vi "PK camera tester CW viewer (frame trigger optional).vi"() -> ()   [LabVIEW 2018]
uses:
  <vilib>/userdefined/High Color/IMAQdx.ctl
  <vilib>/vision/driver/IMAQdx.llb/IMAQdx Attribute Type.ctl
  <vilib>/vision/driver/IMAQdx.llb/IMAQdx Buffer Number Mode.ctl
  convert 1D image array to 2D image - U8 input.vi
  <vilib>/Utility/file.llb/Write Delimited Spreadsheet (I64).vi
  <vilib>/vision/driver/NI_Vision_Acquisition_Software.lvlib
  <resource>/objmgr/imaqdx.rc
  <vilib>/vision/NI_Vision_Development_Module.lvlib
panel:
  out "frame time (s)":dbl format="%#_8g"
  out "frame rate (Hz)":dbl
  in  "stop":bool
  in  "filename":string="myImage"
  in  "path":path=path "C:/Users/QDM2exp/Documents/PK/LabView dev/pk camera stuff"
  in  "save?":bool
  out "max value":u8=131
  in  "external frame start triggers?":bool
  in  "Offset Y":i64(slide) min=0 max=1196 step=4 scale=0.0..1196.0
  in  "Offset X":i64(slide) min=0 max=1916 step=4 scale=0.0..1916.0
  in  "Width":i64(slide)=1920 min=0 max=1920 step=4 scale=0.0..1920.0
  in  "Height":i64(slide)=1200 min=0 max=1200 step=4 scale=0.0..1200.0
  out "Intensity Graph":u8[][](graph)
  in  "Exposure time (us)":dbl=6000.0 min=40.0 max=3000.0 step=1.0
  out "Attribute Information Array":T2(array[cluster])=[{"Attribute Type"=enum."U32", "Readable"=TRUE, "Writable"=TRUE, "Attribute Name"="AcquisitionAttributes::AdvancedGenicam::CommandTimeout"}, {"Attribute Type"=enum."U32", "Readable"=TRUE, "Writable"=TRUE, "Attribute Name"="AcquisitionAttributes::AdvancedGenicam::EventQueueDepth"}, {"Attribute Type"=enum."Bool", "Readable"=TRUE, "Writable"=TRUE, "Attribute Name"="AcquisitionAttributes::AdvancedGenicam::EventsEnabled"}, {"Attribute Type"=enum."Bool", "Readable"=TRUE, "Writable"=FALSE, "Attribute Name"="AcquisitionAttributes::AdvancedGenicam::EventsSupported"}, {"Attribute Type"=enum."Bool", "Readable"=TRUE, "Writable"=TRUE, "Attribute Name"="AcquisitionAttributes::AdvancedGenicam::IgnoreCameraValidationErrors"}, {"Attribute Type"=enum."U32", "Readable"=TRUE, "Writable"=FALSE, "Attribute Name"="AcquisitionAttributes::AdvancedUSB3Vision::ActualMaximumPayloadTransferSize"}, {"Attribute Type"=enum."U32", "Readable"=TRUE, "Writable"=FALSE, "Attribute Name"="AcquisitionAttributes::AdvancedUSB3Vision::RequiredPayloadSizeAlignment"}, {"Attribute Type"=enum."Enum", "Readable"=TRUE, "Writable"=TRUE, "Attribute Name"="AcquisitionAttributes::Bayer::Algorithm"}, {"Attribute Type"=enum."DBL", "Readable"=TRUE, "Writable"=TRUE, "Attribute Name"="AcquisitionAttributes::Bayer::GainB"}, {"Attribute Type"=enum."DBL", "Readable"=TRUE, "Writable"=TRUE, "Attribute Name"="AcquisitionAttributes::Bayer::GainG"}, {"Attribute Type"=enum."DBL", "Readable"=TRUE, "Writable"=TRUE, "Attribute Name"="AcquisitionAttributes::Bayer::GainR"}, {"Attribute Type"=enum."Enum", "Readable"=TRUE, "Writable"=TRUE, "Attribute Name"="AcquisitionAttributes::Bayer::Pattern"}, {"Attribute Type"=enum."Bool", "Readable"=TRUE, "Writable"=TRUE, "Attribute Name"="AcquisitionAttributes::ChunkDataDecoding::ChunkDataDecodingEnabled"}, {"Attribute Type"=enum."U32", "Readable"=TRUE, "Writable"=TRUE, "Attribute Name"="AcquisitionAttributes::ChunkDataDecoding::MaximumChunkCopySize"}, {"Attribute Type"=enum."Enum", "Readable"=TRUE, "Writable"=TRUE, "Attribute Name"="CameraAttributes::SequencerControl::SequencerMode"}, {"Attribute Type"=enum."I64", "Readable"=FALSE, "Writable"=FALSE, "Attribute Name"="CameraAttributes::SequencerControl::SequencerSetActive"}, {"Attribute Type"=enum."Enum", "Readable"=TRUE, "Writable"=TRUE, "Attribute Name"="CameraAttributes::SequencerControl::SequencerConfigurationMode"}, {"Attribute Type"=enum."I64", "Readable"=TRUE, "Writable"=FALSE, "Attribute Name"="CameraAttributes::SequencerControl::SequencerSetStart"}, {"Attribute Type"=enum."I64", "Readable"=TRUE, "Writable"=FALSE, "Attribute Name"="CameraAttributes::SequencerControl::SequencerSetSelector"}, {"Attribute Type"=enum."Command", "Readable"=FALSE, "Writable"=FALSE, "Attribute Name"="CameraAttributes::SequencerControl::SequencerSetLoad"}, {"Attribute Type"=enum."Command", "Readable"=FALSE, "Writable"=FALSE, "Attribute Name"="CameraAttributes::SequencerControl::SequencerSetSave"}, {"Attribute Type"=enum."I64", "Readable"=TRUE, "Writable"=FALSE, "Attribute Name"="CameraAttributes::SequencerControl::SequencerPathSelector"}, {"Attribute Type"=enum."I64", "Readable"=TRUE, "Writable"=FALSE, "Attribute Name"="CameraAttributes::SequencerControl::SequencerSetNext"}, {"Attribute Type"=enum."Enum", "Readable"=TRUE, "Writable"=FALSE, "Attribute Name"="CameraAttributes::SequencerControl::SequencerTriggerSource"}, {"Attribute Type"=enum."Enum", "Readable"=TRUE, "Writable"=FALSE, "Attribute Name"="CameraAttributes::SequencerControl::SequencerTriggerActivation"}, {"Attribute Type"=enum."I64", "Readable"=TRUE, "Writable"=FALSE, "Attribute Name"="CameraAttributes::ImageFormatControl::SensorWidth"}, {"Attribute Type"=enum."I64", "Readable"=TRUE, "Writable"=FALSE, "Attribute Name"="CameraAttributes::ImageFormatControl::SensorHeight"}, {"Attribute Type"=enum."I64", "Readable"=TRUE, "Writable"=FALSE, "Attribute Name"="CameraAttributes::ImageFormatControl::WidthMax"}, {"Attribute Type"=enum."I64", "Readable"=TRUE, "Writable"=FALSE, "Attribute Name"="CameraAttributes::ImageFormatControl::HeightMax"}, {"Attribute Type"=enum."I64", "Readable"=TRUE, "Writable"=TRUE, "Attribute Name"="CameraAttributes::ImageFormatControl::Width"}, {"Attribute Type"=enum."I64", "Readable"=TRUE, "Writable"=TRUE, "Attribute Name"="CameraAttributes::ImageFormatControl::Height"}, {"Attribute Type"=enum."I64", "Readable"=TRUE, "Writable"=TRUE, "Attribute Name"="CameraAttributes::ImageFormatControl::OffsetX"}, {"Attribute Type"=enum."I64", "Readable"=TRUE, "Writable"=TRUE, "Attribute Name"="CameraAttributes::ImageFormatControl::OffsetY"}, {"Attribute Type"=enum."Bool", "Readable"=TRUE, "Writable"=TRUE, "Attribute Name"="CameraAttributes::ImageFormatControl::CenterX"}, {"Attribute Type"=enum."Bool", "Readable"=TRUE, "Writable"=TRUE, "Attribute Name"="CameraAttributes::ImageFormatControl::CenterY"}, {"Attribute Type"=enum."Enum", "Readable"=TRUE, "Writable"=TRUE, "Attribute Name"="CameraAttributes::ImageFormatControl::BinningHorizontalMode"}, {"Attribute Type"=enum."I64", "Readable"=TRUE, "Writable"=TRUE, "Attribute Name"="CameraAttributes::ImageFormatControl::BinningHorizontal"}, {"Attribute Type"=enum."Enum", "Readable"=TRUE, "Writable"=TRUE, "Attribute Name"="CameraAttributes::ImageFormatControl::BinningVerticalMode"}, {"Attribute Type"=enum."I64", "Readable"=TRUE, "Writable"=TRUE, "Attribute Name"="CameraAttributes::ImageFormatControl::BinningVertical"}, {"Attribute Type"=enum."Bool", "Readable"=TRUE, "Writable"=TRUE, "Attribute Name"="CameraAttributes::ImageFormatControl::ReverseX"}, {"Attribute Type"=enum."Bool", "Readable"=TRUE, "Writable"=TRUE, "Attribute Name"="CameraAttributes::ImageFormatControl::ReverseY"}, {"Attribute Type"=enum."Enum", "Readable"=TRUE, "Writable"=TRUE, "Attribute Name"="CameraAttributes::ImageFormatControl::PixelFormat"}, {"Attribute Type"=enum."Enum", "Readable"=TRUE, "Writable"=FALSE, "Attribute Name"="CameraAttributes::ImageFormatControl::PixelSize"}, {"Attribute Type"=enum."Enum", "Readable"=TRUE, "Writable"=FALSE, "Attribute Name"="CameraAttributes::ImageFormatControl::PixelColorFilter"}, {"Attribute Type"=enum."I64", "Readable"=TRUE, "Writable"=FALSE, "Attribute Name"="CameraAttributes::ImageFormatControl::PixelDynamicRangeMin"}, {"Attribute Type"=enum."I64", "Readable"=TRUE, "Writable"=FALSE, "Attribute Name"="CameraAttributes::ImageFormatControl::PixelDynamicRangeMax"}, {"Attribute Type"=enum."Enum", "Readable"=TRUE, "Writable"=TRUE, "Attribute Name"="CameraAttributes::ImageFormatControl::TestImageSelector"}, {"Attribute Type"=enum."Bool", "Readable"=TRUE, "Writable"=TRUE, "Attribute Name"="CameraAttributes::ImageFormatControl::TestImageResetAndHold"}, {"Attribute Type"=enum."Enum", "Readable"=TRUE, "Writable"=TRUE, "Attribute Name"="CameraAttributes::AnalogControl::GainAuto"}, {"Attribute Type"=enum."Enum", "Readable"=TRUE, "Writable"=TRUE, "Attribute Name"="CameraAttributes::AnalogControl::GainSelector"}, {"Attribute Type"=enum."DBL", "Readable"=TRUE, "Writable"=TRUE, "Attribute Name"="CameraAttributes::AnalogControl::Gain"}, {"Attribute Type"=enum."Enum", "Readable"=TRUE, "Writable"=TRUE, "Attribute Name"="CameraAttributes::AnalogControl::BlackLevelSelector"}, {"Attribute Type"=enum."DBL", "Readable"=TRUE, "Writable"=TRUE, "Attribute Name"="CameraAttributes::AnalogControl::BlackLevel"}, {"Attribute Type"=enum."DBL", "Readable"=TRUE, "Writable"=TRUE, "Attribute Name"="CameraAttributes::AnalogControl::Gamma"}, {"Attribute Type"=enum."I64", "Readable"=TRUE, "Writable"=TRUE, "Attribute Name"="CameraAttributes::AnalogControl::DigitalShift"}, {"Attribute Type"=enum."DBL", "Readable"=FALSE, "Writable"=FALSE, "Attribute Name"="CameraAttributes::ImageQualityControl::ColorTransformationValue"}, {"Attribute Type"=enum."Enum", "Readable"=TRUE, "Writable"=TRUE, "Attribute Name"="CameraAttributes::AcquisitionControl::AcquisitionMode"}, {"Attribute Type"=enum."Enum", "Readable"=TRUE, "Writable"=TRUE, "Attribute Name"="CameraAttributes::AcquisitionControl::ShutterMode"}, {"Attribute Type"=enum."Enum", "Readable"=TRUE, "Writable"=TRUE, "Attribute Name"="CameraAttributes::AcquisitionControl::ExposureAuto"}, {"Attribute Type"=enum."Enum", "Readable"=TRUE, "Writable"=TRUE, "Attribute Name"="CameraAttributes::AcquisitionControl::ExposureMode"}, {"Attribute Type"=enum."DBL", "Readable"=TRUE, "Writable"=TRUE, "Attribute Name"="CameraAttributes::AcquisitionControl::ExposureTime"}, {"Attribute Type"=enum."Enum", "Readable"=FALSE, "Writable"=FALSE, "Attribute Name"="CameraAttributes::AcquisitionControl::ExposureOverlapTimeMode"}, {"Attribute Type"=enum."DBL", "Readable"=FALSE, "Writable"=FALSE, "Attribute Name"="CameraAttributes::AcquisitionControl::ExposureOverlapTimeMax"}, {"Attribute Type"=enum."I64", "Readable"=TRUE, "Writable"=TRUE, "Attribute Name"="CameraAttributes::AcquisitionControl::AcquisitionBurstFrameCount"}, {"Attribute Type"=enum."Enum", "Readable"=TRUE, "Writable"=TRUE, "Attribute Name"="CameraAttributes::AcquisitionControl::TriggerSelector"}, {"Attribute Type"=enum."Enum", "Readable"=TRUE, "Writable"=TRUE, "Attribute Name"="CameraAttributes::AcquisitionControl::TriggerMode"}, {"Attribute Type"=enum."Command", "Readable"=FALSE, "Writable"=TRUE, "Attribute Name"="CameraAttributes::AcquisitionControl::TriggerSoftware"}, {"Attribute Type"=enum."Enum", "Readable"=TRUE, "Writable"=TRUE, "Attribute Name"="CameraAttributes::AcquisitionControl::TriggerSource"}, {"Attribute Type"=enum."Enum", "Readable"=TRUE, "Writable"=TRUE, "Attribute Name"="CameraAttributes::AcquisitionControl::TriggerActivation"}, {"Attribute Type"=enum."DBL", "Readable"=TRUE, "Writable"=TRUE, "Attribute Name"="CameraAttributes::AcquisitionControl::TriggerDelay"}, {"Attribute Type"=enum."Bool", "Readable"=TRUE, "Writable"=TRUE, "Attribute Name"="CameraAttributes::AcquisitionControl::AcquisitionFrameRateEnable"}, {"Attribute Type"=enum."DBL", "Readable"=TRUE, "Writable"=TRUE, "Attribute Name"="CameraAttributes::AcquisitionControl::AcquisitionFrameRate"}, {"Attribute Type"=enum."DBL", "Readable"=TRUE, "Writable"=FALSE, "Attribute Name"="CameraAttributes::AcquisitionControl::ResultingFrameRate"}, {"Attribute Type"=enum."DBL", "Readable"=TRUE, "Writable"=FALSE, "Attribute Name"="CameraAttributes::AcquisitionControl::SensorReadoutTime"}, {"Attribute Type"=enum."Enum", "Readable"=TRUE, "Writable"=TRUE, "Attribute Name"="CameraAttributes::AcquisitionControl::AcquisitionStatusSelector"}, {"Attribute Type"=enum."Bool", "Readable"=TRUE, "Writable"=FALSE, "Attribute Name"="CameraAttributes::AcquisitionControl::AcquisitionStatus"}, {"Attribute Type"=enum."DBL", "Readable"=TRUE, "Writable"=TRUE, "Attribute Name"="CameraAttributes::AutoFunctionControl::AutoTargetBrightness"}, {"Attribute Type"=enum."Enum", "Readable"=TRUE, "Writable"=TRUE, "Attribute Name"="CameraAttributes::AutoFunctionControl::AutoFunctionProfile"}, {"Attribute Type"=enum."DBL", "Readable"=TRUE, "Writable"=TRUE, "Attribute Name"="CameraAttributes::AutoFunctionControl::AutoGainLowerLimit"}, {"Attribute Type"=enum."DBL", "Readable"=TRUE, "Writable"=TRUE, "Attribute Name"="CameraAttributes::AutoFunctionControl::AutoGainUpperLimit"}, {"Attribute Type"=enum."DBL", "Readable"=TRUE, "Writable"=TRUE, "Attribute Name"="CameraAttributes::AutoFunctionControl::AutoExposureTimeLowerLimit"}, {"Attribute Type"=enum."DBL", "Readable"=TRUE, "Writable"=TRUE, "Attribute Name"="CameraAttributes::AutoFunctionControl::AutoExposureTimeUpperLimit"}, {"Attribute Type"=enum."Enum", "Readable"=TRUE, "Writable"=TRUE, "Attribute Name"="CameraAttributes::AutoFunctionControl::AutoFunctionROIControl::AutoFunctionROISelector"}, {"Attribute Type"=enum."I64", "Readable"=TRUE, "Writable"=TRUE, "Attribute Name"="CameraAttributes::AutoFunctionControl::AutoFunctionROIControl::AutoFunctionROIWidth"}, {"Attribute Type"=enum."I64", "Readable"=TRUE, "Writable"=TRUE, "Attribute Name"="CameraAttributes::AutoFunctionControl::AutoFunctionROIControl::AutoFunctionROIHeight"}, {"Attribute Type"=enum."I64", "Readable"=TRUE, "Writable"=TRUE, "Attribute Name"="CameraAttributes::AutoFunctionControl::AutoFunctionROIControl::AutoFunctionROIOffsetX"}, {"Attribute Type"=enum."I64", "Readable"=TRUE, "Writable"=TRUE, "Attribute Name"="CameraAttributes::AutoFunctionControl::AutoFunctionROIControl::AutoFunctionROIOffsetY"}, {"Attribute Type"=enum."Bool", "Readable"=TRUE, "Writable"=TRUE, "Attribute Name"="CameraAttributes::AutoFunctionControl::AutoFunctionROIControl::AutoFunctionROIUseBrightness"}, {"Attribute Type"=enum."Bool", "Readable"=TRUE, "Writable"=TRUE, "Attribute Name"="CameraAttributes::AutoFunctionControl::AutoFunctionROIControl::AutoFunctionROIUseWhiteBalance"}, {"Attribute Type"=enum."Enum", "Readable"=TRUE, "Writable"=TRUE, "Attribute Name"="CameraAttributes::LUTControl::LUTSelector"}, {"Attribute Type"=enum."Bool", "Readable"=TRUE, "Writable"=TRUE, "Attribute Name"="CameraAttributes::LUTControl::LUTEnable"}, {"Attribute Type"=enum."I64", "Readable"=TRUE, "Writable"=TRUE, "Attribute Name"="CameraAttributes::LUTControl::LUTIndex"}, {"Attribute Type"=enum."I64", "Readable"=TRUE, "Writable"=TRUE, "Attribute Name"="CameraAttributes::LUTControl::LUTValue"}, {"Attribute Type"=enum."Enum", "Readable"=TRUE, "Writable"=TRUE, "Attribute Name"="CameraAttributes::DigitalIOControl::LineSelector"}, {"Attribute Type"=enum."Enum", "Readable"=TRUE, "Writable"=TRUE, "Attribute Name"="CameraAttributes::DigitalIOControl::LineMode"}, {"Attribute Type"=enum."Enum", "Readable"=TRUE, "Writable"=FALSE, "Attribute Name"="CameraAttributes::DigitalIOControl::LineFormat"}, {"Attribute Type"=enum."Enum", "Readable"=TRUE, "Writable"=FALSE, "Attribute Name"="CameraAttributes::DigitalIOControl::LineLogic"}, {"Attribute Type"=enum."Enum", "Readable"=FALSE, "Writable"=FALSE, "Attribute Name"="CameraAttributes::DigitalIOControl::LineSource"}, {"Attribute Type"=enum."Bool", "Readable"=TRUE, "Writable"=TRUE, "Attribute Name"="CameraAttributes::DigitalIOControl::LineInverter"}, {"Attribute Type"=enum."DBL", "Readable"=TRUE, "Writable"=TRUE, "Attribute Name"="CameraAttributes::DigitalIOControl::LineDebouncerTime"}, {"Attribute Type"=enum."DBL", "Readable"=FALSE, "Writable"=FALSE, "Attribute Name"="CameraAttributes::DigitalIOControl::LineMinimumOutputPulseWidth"}, {"Attribute Type"=enum."Bool", "Readable"=FALSE, "Writable"=FALSE, "Attribute Name"="CameraAttributes::DigitalIOControl::LineOverloadStatus"}, {"Attribute Type"=enum."Bool", "Readable"=TRUE, "Writable"=FALSE, "Attribute Name"="CameraAttributes::DigitalIOControl::LineStatus"}, {"Attribute Type"=enum."I64", "Readable"=TRUE, "Writable"=FALSE, "Attribute Name"="CameraAttributes::DigitalIOControl::LineStatusAll"}, {"Attribute Type"=enum."Enum", "Readable"=TRUE, "Writable"=TRUE, "Attribute Name"="CameraAttributes::DigitalIOControl::UserOutputSelector"}, {"Attribute Type"=enum."Bool", "Readable"=TRUE, "Writable"=TRUE, "Attribute Name"="CameraAttributes::DigitalIOControl::UserOutputValue"}, {"Attribute Type"=enum."I64", "Readable"=TRUE, "Writable"=TRUE, "Attribute Name"="CameraAttributes::DigitalIOControl::UserOutputValueAll"}, {"Attribute Type"=enum."Enum", "Readable"=TRUE, "Writable"=TRUE, "Attribute Name"="CameraAttributes::SoftwareSignalControl::SoftwareSignalSelector"}, {"Attribute Type"=enum."Command", "Readable"=FALSE, "Writable"=TRUE, "Attribute Name"="CameraAttributes::SoftwareSignalControl::SoftwareSignalPulse"}, {"Attribute Type"=enum."Enum", "Readable"=TRUE, "Writable"=TRUE, "Attribute Name"="CameraAttributes::CounterAndTimerControl::TimerSelector"}, {"Attribute Type"=enum."DBL", "Readable"=TRUE, "Writable"=TRUE, "Attribute Name"="CameraAttributes::CounterAndTimerControl::TimerDuration"}, {"Attribute Type"=enum."DBL", "Readable"=TRUE, "Writable"=TRUE, "Attribute Name"="CameraAttributes::CounterAndTimerControl::TimerDelay"}, {"Attribute Type"=enum."Enum", "Readable"=TRUE, "Writable"=TRUE, "Attribute Name"="CameraAttributes::CounterAndTimerControl::TimerTriggerSource"}, {"Attribute Type"=enum."Enum", "Readable"=TRUE, "Writable"=TRUE, "Attribute Name"="CameraAttributes::CounterAndTimerControl::CounterSelector"}, {"Attribute Type"=enum."Enum", "Readable"=TRUE, "Writable"=TRUE, "Attribute Name"="CameraAttributes::CounterAndTimerControl::CounterEventSource"}, {"Attribute Type"=enum."Enum", "Readable"=TRUE, "Writable"=TRUE, "Attribute Name"="CameraAttributes::CounterAndTimerControl::CounterResetSource"}, {"Attribute Type"=enum."Enum", "Readable"=TRUE, "Writable"=TRUE, "Attribute Name"="CameraAttributes::CounterAndTimerControl::CounterResetActivation"}, {"Attribute Type"=enum."Command", "Readable"=FALSE, "Writable"=FALSE, "Attribute Name"="CameraAttributes::CounterAndTimerControl::CounterReset"}, {"Attribute Type"=enum."I64", "Readable"=TRUE, "Writable"=TRUE, "Attribute Name"="CameraAttributes::CounterAndTimerControl::CounterDuration"}, {"Attribute Type"=enum."Bool", "Readable"=TRUE, "Writable"=TRUE, "Attribute Name"="CameraAttributes::ChunkDataControl::ChunkModeActive"}, {"Attribute Type"=enum."Enum", "Readable"=TRUE, "Writable"=TRUE, "Attribute Name"="CameraAttributes::ChunkDataControl::ChunkSelector"}, {"Attribute Type"=enum."Bool", "Readable"=TRUE, "Writable"=TRUE, "Attribute Name"="CameraAttributes::ChunkDataControl::ChunkEnable"}, {"Attribute Type"=enum."Enum", "Readable"=FALSE, "Writable"=FALSE, "Attribute Name"="CameraAttributes::ChunkDataControl::ChunkGainSelector"}, {"Attribute Type"=enum."DBL", "Readable"=FALSE, "Writable"=FALSE, "Attribute Name"="CameraAttributes::ChunkDataControl::ChunkGain"}, {"Attribute Type"=enum."DBL", "Readable"=FALSE, "Writable"=FALSE, "Attribute Name"="CameraAttributes::ChunkDataControl::ChunkExposureTime"}, {"Attribute Type"=enum."I64", "Readable"=FALSE, "Writable"=FALSE, "Attribute Name"="CameraAttributes::ChunkDataControl::ChunkTimestamp"}, {"Attribute Type"=enum."I64", "Readable"=FALSE, "Writable"=FALSE, "Attribute Name"="CameraAttributes::ChunkDataControl::ChunkLineStatusAll"}, {"Attribute Type"=enum."Enum", "Readable"=FALSE, "Writable"=FALSE, "Attribute Name"="CameraAttributes::ChunkDataControl::ChunkCounterSelector"}, {"Attribute Type"=enum."I64", "Readable"=FALSE, "Writable"=FALSE, "Attribute Name"="CameraAttributes::ChunkDataControl::ChunkCounterValue"}, {"Attribute Type"=enum."I64", "Readable"=FALSE, "Writable"=FALSE, "Attribute Name"="CameraAttributes::ChunkDataControl::ChunkSequencerSetActive"}, {"Attribute Type"=enum."I64", "Readable"=FALSE, "Writable"=FALSE, "Attribute Name"="CameraAttributes::ChunkDataControl::ChunkPayloadCRC16"}, {"Attribute Type"=enum."Enum", "Readable"=FALSE, "Writable"=FALSE, "Attribute Name"="CameraAttributes::ChunkDataControl::ChunkData::ChunkGainSelector"}, {"Attribute Type"=enum."DBL", "Readable"=FALSE, "Writable"=FALSE, "Attribute Name"="CameraAttributes::ChunkDataControl::ChunkData::ChunkGain"}, {"Attribute Type"=enum."DBL", "Readable"=FALSE, "Writable"=FALSE, "Attribute Name"="CameraAttributes::ChunkDataControl::ChunkData::ChunkExposureTime"}, {"Attribute Type"=enum."I64", "Readable"=FALSE, "Writable"=FALSE, "Attribute Name"="CameraAttributes::ChunkDataControl::ChunkData::ChunkTimestamp"}, {"Attribute Type"=enum."I64", "Readable"=FALSE, "Writable"=FALSE, "Attribute Name"="CameraAttributes::ChunkDataControl::ChunkData::ChunkLineStatusAll"}, {"Attribute Type"=enum."Enum", "Readable"=FALSE, "Writable"=FALSE, "Attribute Name"="CameraAttributes::ChunkDataControl::ChunkData::ChunkCounterSelector"}, {"Attribute Type"=enum."I64", "Readable"=FALSE, "Writable"=FALSE, "Attribute Name"="CameraAttributes::ChunkDataControl::ChunkData::ChunkCounterValue"}, {"Attribute Type"=enum."I64", "Readable"=FALSE, "Writable"=FALSE, "Attribute Name"="CameraAttributes::ChunkDataControl::ChunkData::ChunkSequencerSetActive"}, {"Attribute Type"=enum."I64", "Readable"=FALSE, "Writable"=FALSE, "Attribute Name"="CameraAttributes::ChunkDataControl::ChunkData::ChunkPayloadCRC16"}, {"Attribute Type"=enum."Enum", "Readable"=TRUE, "Writable"=TRUE, "Attribute Name"="CameraAttributes::EventControl::EventSelector"}, {"Attribute Type"=enum."Enum", "Readable"=TRUE, "Writable"=TRUE, "Attribute Name"="CameraAttributes::EventControl::EventNotification"}, {"Attribute Type"=enum."I64", "Readable"=FALSE, "Writable"=FALSE, "Attribute Name"="CameraAttributes::EventControl::EventExposureEndData::EventExposureEnd"}, {"Attribute Type"=enum."I64", "Readable"=FALSE, "Writable"=FALSE, "Attribute Name"="CameraAttributes::EventControl::EventExposureEndData::EventExposureEndTimestamp"}, {"Attribute Type"=enum."I64", "Readable"=FALSE, "Writable"=FALSE, "Attribute Name"="CameraAttributes::EventControl::EventExposureEndData::EventExposureEndFrameID"}, {"Attribute Type"=enum."I64", "Readable"=FALSE, "Writable"=FALSE, "Attribute Name"="CameraAttributes::EventControl::EventFrameStartData::EventFrameStart"}, {"Attribute Type"=enum."I64", "Readable"=FALSE, "Writable"=FALSE, "Attribute Name"="CameraAttributes::EventControl::EventFrameStartData::EventFrameStartTimestamp"}, {"Attribute Type"=enum."I64", "Readable"=FALSE, "Writable"=FALSE, "Attribute Name"="CameraAttributes::EventControl::EventFrameStartData::EventFrameStartFrameID"}, {"Attribute Type"=enum."I64", "Readable"=FALSE, "Writable"=FALSE, "Attribute Name"="CameraAttributes::EventControl::EventFrameBurstStartData::EventFrameBurstStart"}, {"Attribute Type"=enum."I64", "Readable"=FALSE, "Writable"=FALSE, "Attribute Name"="CameraAttributes::EventControl::EventFrameBurstStartData::EventFrameBurstStartTimestamp"}, {"Attribute Type"=enum."I64", "Readable"=FALSE, "Writable"=FALSE, "Attribute Name"="CameraAttributes::EventControl::EventFrameBurstStartData::EventFrameBurstStartFrameID"}, {"Attribute Type"=enum."I64", "Readable"=FALSE, "Writable"=FALSE, "Attribute Name"="CameraAttributes::EventControl::EventFrameStartOvertriggerData::EventFrameStartOvertrigger"}, {"Attribute Type"=enum."I64", "Readable"=FALSE, "Writable"=FALSE, "Attribute Name"="CameraAttributes::EventControl::EventFrameStartOvertriggerData::EventFrameStartOvertriggerTimestamp"}, {"Attribute Type"=enum."I64", "Readable"=FALSE, "Writable"=FALSE, "Attribute Name"="CameraAttributes::EventControl::EventFrameStartOvertriggerData::EventFrameStartOvertriggerFrameID"}, {"Attribute Type"=enum."I64", "Readable"=FALSE, "Writable"=FALSE, "Attribute Name"="CameraAttributes::EventControl::EventFrameBurstStartOvertriggerData::EventFrameBurstStartOvertrigger"}, {"Attribute Type"=enum."I64", "Readable"=FALSE, "Writable"=FALSE, "Attribute Name"="CameraAttributes::EventControl::EventFrameBurstStartOvertriggerData::EventFrameBurstStartOvertriggerTimestamp"}, {"Attribute Type"=enum."I64", "Readable"=FALSE, "Writable"=FALSE, "Attribute Name"="CameraAttributes::EventControl::EventFrameBurstStartOvertriggerData::EventFrameBurstStartOvertriggerFrameID"}, {"Attribute Type"=enum."I64", "Readable"=FALSE, "Writable"=FALSE, "Attribute Name"="CameraAttributes::EventControl::EventCriticalTemperatureData::EventCriticalTemperature"}, {"Attribute Type"=enum."I64", "Readable"=FALSE, "Writable"=FALSE, "Attribute Name"="CameraAttributes::EventControl::EventCriticalTemperatureData::EventCriticalTemperatureTimestamp"}, {"Attribute Type"=enum."I64", "Readable"=FALSE, "Writable"=FALSE, "Attribute Name"="CameraAttributes::EventControl::EventOverTemperatureData::EventOverTemperature"}, {"Attribute Type"=enum."I64", "Readable"=FALSE, "Writable"=FALSE, "Attribute Name"="CameraAttributes::EventControl::EventOverTemperatureData::EventOverTemperatureTimestamp"}, {"Attribute Type"=enum."I64", "Readable"=FALSE, "Writable"=FALSE, "Attribute Name"="CameraAttributes::EventControl::EventFrameStartWaitData::EventFrameStartWait"}, {"Attribute Type"=enum."I64", "Readable"=FALSE, "Writable"=FALSE, "Attribute Name"="CameraAttributes::EventControl::EventFrameStartWaitData::EventFrameStartWaitTimestamp"}, {"Attribute Type"=enum."I64", "Readable"=FALSE, "Writable"=FALSE, "Attribute Name"="CameraAttributes::EventControl::EventFrameBurstStartWaitData::EventFrameBurstStartWait"}, {"Attribute Type"=enum."I64", "Readable"=FALSE, "Writable"=FALSE, "Attribute Name"="CameraAttributes::EventControl::EventFrameBurstStartWaitData::EventFrameBurstStartWaitTimestamp"}, {"Attribute Type"=enum."Enum", "Readable"=TRUE, "Writable"=TRUE, "Attribute Name"="CameraAttributes::UserSetControl::UserSetSelector"}, {"Attribute Type"=enum."Command", "Readable"=FALSE, "Writable"=TRUE, "Attribute Name"="CameraAttributes::UserSetControl::UserSetLoad"}, {"Attribute Type"=enum."Command", "Readable"=FALSE, "Writable"=TRUE, "Attribute Name"="CameraAttributes::UserSetControl::UserSetSave"}, {"Attribute Type"=enum."Enum", "Readable"=TRUE, "Writable"=TRUE, "Attribute Name"="CameraAttributes::UserSetControl::UserSetDefault"}, {"Attribute Type"=enum."I64", "Readable"=TRUE, "Writable"=FALSE, "Attribute Name"="CameraAttributes::TransportLayerControl::PayloadSize"}, {"Attribute Type"=enum."Enum", "Readable"=TRUE, "Writable"=FALSE, "Attribute Name"="CameraAttributes::TransportLayerControl::BslUSBSpeedMode"}, {"Attribute Type"=enum."I64", "Readable"=TRUE, "Writable"=FALSE, "Attribute Name"="CameraAttributes::TransportLayerControl::SIPayloadTransferSize"}, {"Attribute Type"=enum."I64", "Readable"=TRUE, "Writable"=FALSE, "Attribute Name"="CameraAttributes::TransportLayerControl::SIPayloadTransferCount"}, {"Attribute Type"=enum."I64", "Readable"=TRUE, "Writable"=FALSE, "Attribute Name"="CameraAttributes::TransportLayerControl::SIPayloadFinalTransfer1Size"}, {"Attribute Type"=enum."I64", "Readable"=TRUE, "Writable"=FALSE, "Attribute Name"="CameraAttributes::TransportLayerControl::SIPayloadFinalTransfer2Size"}, {"Attribute Type"=enum."String", "Readable"=TRUE, "Writable"=FALSE, "Attribute Name"="CameraAttributes::DeviceControl::DeviceVendorName"}, {"Attribute Type"=enum."String", "Readable"=TRUE, "Writable"=FALSE, "Attribute Name"="CameraAttributes::DeviceControl::DeviceModelName"}, {"Attribute Type"=enum."String", "Readable"=TRUE, "Writable"=FALSE, "Attribute Name"="CameraAttributes::DeviceControl::DeviceManufacturerInfo"}, {"Attribute Type"=enum."String", "Readable"=TRUE, "Writable"=FALSE, "Attribute Name"="CameraAttributes::DeviceControl::DeviceVersion"}, {"Attribute Type"=enum."String", "Readable"=TRUE, "Writable"=FALSE, "Attribute Name"="CameraAttributes::DeviceControl::DeviceFirmwareVersion"}, {"Attribute Type"=enum."String", "Readable"=TRUE, "Writable"=FALSE, "Attribute Name"="CameraAttributes::DeviceControl::DeviceSerialNumber"}, {"Attribute Type"=enum."String", "Readable"=TRUE, "Writable"=TRUE, "Attribute Name"="CameraAttributes::DeviceControl::DeviceUserID"}, {"Attribute Type"=enum."Enum", "Readable"=TRUE, "Writable"=FALSE, "Attribute Name"="CameraAttributes::DeviceControl::DeviceScanType"}, {"Attribute Type"=enum."Command", "Readable"=FALSE, "Writable"=TRUE, "Attribute Name"="CameraAttributes::DeviceControl::TimestampLatch"}, {"Attribute Type"=enum."I64", "Readable"=TRUE, "Writable"=FALSE, "Attribute Name"="CameraAttributes::DeviceControl::TimestampLatchValue"}, {"Attribute Type"=enum."I64", "Readable"=TRUE, "Writable"=TRUE, "Attribute Name"="CameraAttributes::DeviceControl::DeviceLinkSelector"}, {"Attribute Type"=enum."I64", "Readable"=TRUE, "Writable"=FALSE, "Attribute Name"="CameraAttributes::DeviceControl::DeviceLinkSpeed"}, {"Attribute Type"=enum."Enum", "Readable"=TRUE, "Writable"=TRUE, "Attribute Name"="CameraAttributes::DeviceControl::DeviceLinkThroughputLimitMode"}, {"Attribute Type"=enum."I64", "Readable"=TRUE, "Writable"=TRUE, "Attribute Name"="CameraAttributes::DeviceControl::DeviceLinkThroughputLimit"}, {"Attribute Type"=enum."I64", "Readable"=TRUE, "Writable"=FALSE, "Attribute Name"="CameraAttributes::DeviceControl::DeviceLinkCurrentThroughput"}, {"Attribute Type"=enum."Enum", "Readable"=TRUE, "Writable"=TRUE, "Attribute Name"="CameraAttributes::DeviceControl::DeviceTemperatureSelector"}, {"Attribute Type"=enum."DBL", "Readable"=TRUE, "Writable"=FALSE, "Attribute Name"="CameraAttributes::DeviceControl::DeviceTemperature"}, {"Attribute Type"=enum."Enum", "Readable"=TRUE, "Writable"=FALSE, "Attribute Name"="CameraAttributes::DeviceControl::TemperatureState"}, {"Attribute Type"=enum."I64", "Readable"=TRUE, "Writable"=FALSE, "Attribute Name"="CameraAttributes::DeviceControl::DeviceSFNCVersionMajor"}, {"Attribute Type"=enum."I64", "Readable"=TRUE, "Writable"=FALSE, "Attribute Name"="CameraAttributes::DeviceControl::DeviceSFNCVersionMinor"}, {"Attribute Type"=enum."I64", "Readable"=TRUE, "Writable"=FALSE, "Attribute Name"="CameraAttributes::DeviceControl::DeviceSFNCVersionSubMinor"}, {"Attribute Type"=enum."Enum", "Readable"=TRUE, "Writable"=TRUE, "Attribute Name"="CameraAttributes::UserDefinedValueControl::UserDefinedValueSelector"}, {"Attribute Type"=enum."I64", "Readable"=TRUE, "Writable"=TRUE, "Attribute Name"="CameraAttributes::UserDefinedValueControl::UserDefinedValue"}, {"Attribute Type"=enum."Enum", "Readable"=TRUE, "Writable"=TRUE, "Attribute Name"="CameraAttributes::RemoveParameterLimitControl::RemoveParameterLimitSelector"}, {"Attribute Type"=enum."Bool", "Readable"=TRUE, "Writable"=TRUE, "Attribute Name"="CameraAttributes::RemoveParameterLimitControl::RemoveParameterLimit"}, {"Attribute Type"=enum."Enum", "Readable"=TRUE, "Writable"=TRUE, "Attribute Name"="CameraAttributes::ExpertFeatureAccess::ExpertFeatureAccessSelector"}, {"Attribute Type"=enum."I64", "Readable"=TRUE, "Writable"=TRUE, "Attribute Name"="CameraAttributes::ExpertFeatureAccess::ExpertFeatureAccessKey"}, {"Attribute Type"=enum."Bool", "Readable"=FALSE, "Writable"=FALSE, "Attribute Name"="CameraAttributes::ExpertFeatureAccess::ExpertFeatureEnable"}, {"Attribute Type"=enum."Enum", "Readable"=TRUE, "Writable"=TRUE, "Attribute Name"="CameraAttributes::FileAccessControl::FileSelector"}, {"Attribute Type"=enum."Enum", "Readable"=TRUE, "Writable"=TRUE, "Attribute Name"="CameraAttributes::FileAccessControl::FileOperationSelector"}, {"Attribute Type"=enum."Enum", "Readable"=TRUE, "Writable"=TRUE, "Attribute Name"="CameraAttributes::FileAccessControl::FileOpenMode"}, {"Attribute Type"=enum."I64", "Readable"=TRUE, "Writable"=TRUE, "Attribute Name"="CameraAttributes::FileAccessControl::FileAccessOffset"}, {"Attribute Type"=enum."I64", "Readable"=TRUE, "Writable"=TRUE, "Attribute Name"="CameraAttributes::FileAccessControl::FileAccessLength"}, {"Attribute Type"=enum."Enum", "Readable"=TRUE, "Writable"=FALSE, "Attribute Name"="CameraAttributes::FileAccessControl::FileOperationStatus"}, {"Attribute Type"=enum."I64", "Readable"=TRUE, "Writable"=FALSE, "Attribute Name"="CameraAttributes::FileAccessControl::FileOperationResult"}, {"Attribute Type"=enum."I64", "Readable"=TRUE, "Writable"=FALSE, "Attribute Name"="CameraAttributes::FileAccessControl::FileSize"}, {"Attribute Type"=enum."Command", "Readable"=FALSE, "Writable"=TRUE, "Attribute Name"="CameraAttributes::FileAccessControl::FileOperationExecute"}, {"Attribute Type"=enum."Enum", "Readable"=TRUE, "Writable"=TRUE, "Attribute Name"="AcquisitionAttributes::BitsPerPixel"}, {"Attribute Type"=enum."Enum", "Readable"=TRUE, "Writable"=TRUE, "Attribute Name"="AcquisitionAttributes::ImageDecoderCopyMode"}, {"Attribute Type"=enum."Enum", "Readable"=TRUE, "Writable"=TRUE, "Attribute Name"="AcquisitionAttributes::IncompleteBufferMode"}, {"Attribute Type"=enum."Enum", "Readable"=TRUE, "Writable"=TRUE, "Attribute Name"="AcquisitionAttributes::OutputImageType"}, {"Attribute Type"=enum."Enum", "Readable"=TRUE, "Writable"=TRUE, "Attribute Name"="AcquisitionAttributes::OverwriteMode"}, {"Attribute Type"=enum."Enum", "Readable"=TRUE, "Writable"=TRUE, "Attribute Name"="AcquisitionAttributes::ReceiveTimestampMode"}, {"Attribute Type"=enum."Bool", "Readable"=TRUE, "Writable"=TRUE, "Attribute Name"="AcquisitionAttributes::ShiftPixelBits"}, {"Attribute Type"=enum."Bool", "Readable"=TRUE, "Writable"=TRUE, "Attribute Name"="AcquisitionAttributes::SwapPixelBytes"}, {"Attribute Type"=enum."U32", "Readable"=TRUE, "Writable"=TRUE, "Attribute Name"="AcquisitionAttributes::Timeout"}, {"Attribute Type"=enum."U32", "Readable"=TRUE, "Writable"=FALSE, "Attribute Name"="CameraInformation::BaseAddress"}, {"Attribute Type"=enum."Enum", "Readable"=TRUE, "Writable"=FALSE, "Attribute Name"="CameraInformation::BusType"}, {"Attribute Type"=enum."String", "Readable"=TRUE, "Writable"=FALSE, "Attribute Name"="CameraInformation::ModelName"}, {"Attribute Type"=enum."String", "Readable"=TRUE, "Writable"=FALSE, "Attribute Name"="CameraInformation::PrimaryURLString"}, {"Attribute Type"=enum."String", "Readable"=TRUE, "Writable"=FALSE, "Attribute Name"="CameraInformation::SecondaryURLString"}, {"Attribute Type"=enum."U32", "Readable"=TRUE, "Writable"=FALSE, "Attribute Name"="CameraInformation::SerialNumberHigh"}, {"Attribute Type"=enum."U32", "Readable"=TRUE, "Writable"=FALSE, "Attribute Name"="CameraInformation::SerialNumberLow"}, {"Attribute Type"=enum."Enum", "Readable"=TRUE, "Writable"=FALSE, "Attribute Name"="CameraInformation::USBConnectionSpeed"}, {"Attribute Type"=enum."String", "Readable"=TRUE, "Writable"=FALSE, "Attribute Name"="CameraInformation::VendorName"}, {"Attribute Type"=enum."Bool", "Readable"=TRUE, "Writable"=FALSE, "Attribute Name"="StatusInformation::AcqInProgress"}, {"Attribute Type"=enum."I64", "Readable"=TRUE, "Writable"=FALSE, "Attribute Name"="StatusInformation::HandledEventCount"}, {"Attribute Type"=enum."I64", "Readable"=TRUE, "Writable"=FALSE, "Attribute Name"="StatusInformation::IncompleteBufferCount"}, {"Attribute Type"=enum."I64", "Readable"=TRUE, "Writable"=FALSE, "Attribute Name"="StatusInformation::LastBufferCount"}, {"Attribute Type"=enum."U32", "Readable"=TRUE, "Writable"=FALSE, "Attribute Name"="StatusInformation::LastBufferNumber"}, {"Attribute Type"=enum."I64", "Readable"=TRUE, "Writable"=FALSE, "Attribute Name"="StatusInformation::LostBufferCount"}, {"Attribute Type"=enum."I64", "Readable"=TRUE, "Writable"=FALSE, "Attribute Name"="StatusInformation::LostEventCount"}]
  in  "Session In":T3="cam0"
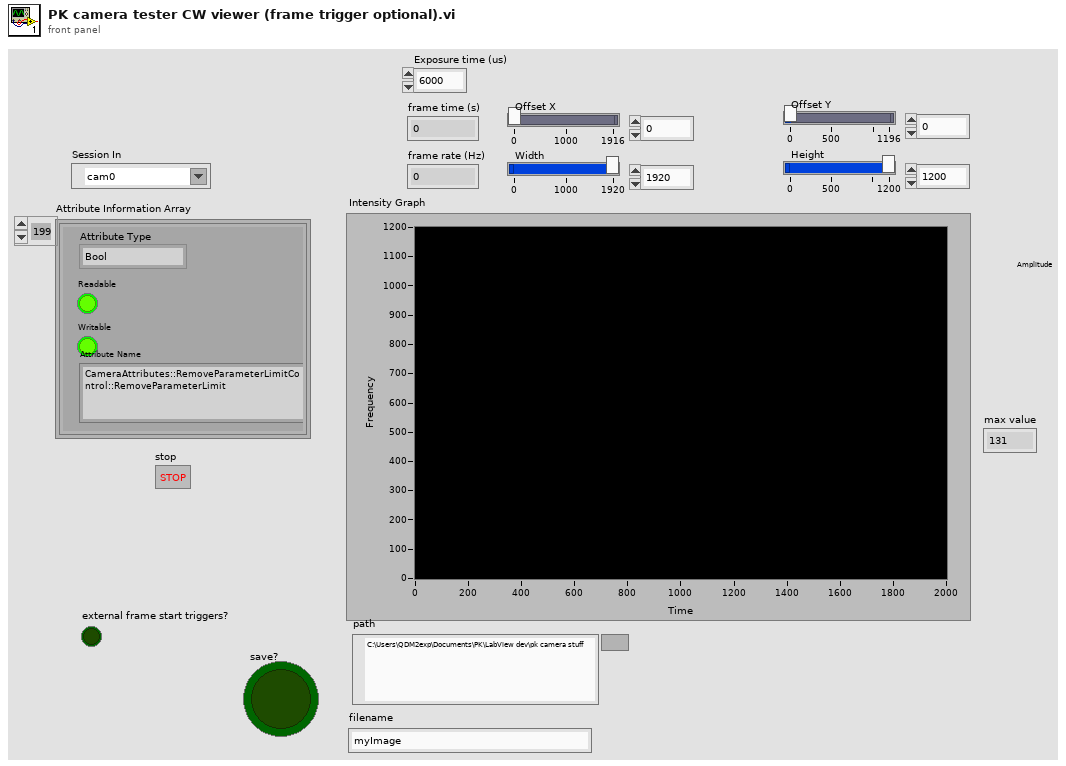
[diagram p1: front panel]
types:
  T1 = typedef "NI_Vision_Acquisition_Software.lvlib/IMAQdx Attribute Type.ctl" = enum32{"U32", "I64", "DBL", "String", "Enum", "Bool", "Command"}
  T2 = cluster{"Attribute Type":T1, "Readable":bool, "Writable":bool, "Attribute Name":string}[]
  T3 = typedef "IMAQdx.ctl" = refnum<k21>
  T4 = typedef "Image Type" = u32
  T5 = typedef "IMAQ Image.ctl" = refnum<image>
  T6 = typedef "NI_Vision_Acquisition_Software.lvlib/IMAQdx Buffer Number Mode.ctl" = enum32{"Next", "Last", "Buffer Number", "Every", "Last New"}
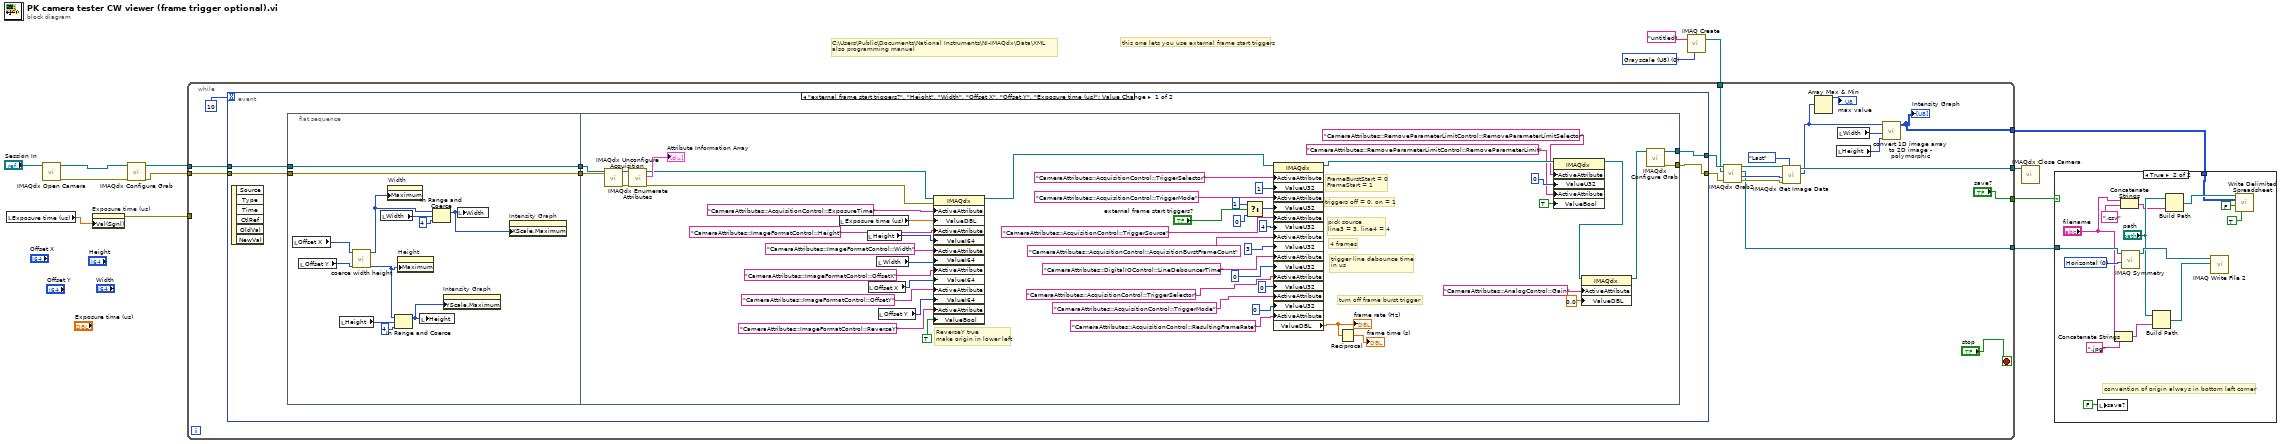
[diagram p0: block diagram]
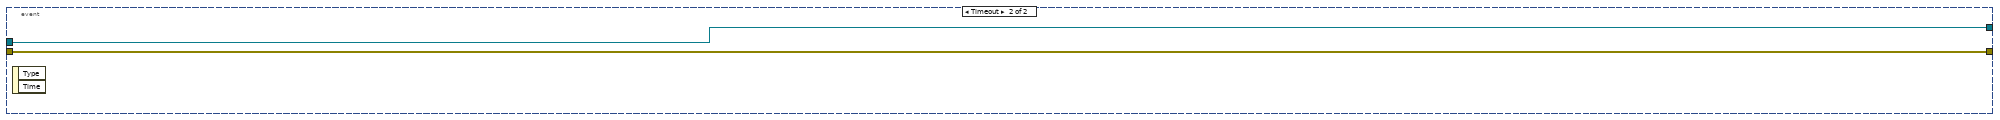
[diagram p3: hidden frame]
diagram:
  w9 = T4 0 items=["Grayscale (U8)", "Grayscale (I16)", "Grayscale (SGL)", "Complex (CSG)", "RGB (U32)", "HSL (U32)", "RGB (U64)", "Grayscale (U16)"] ("Image Type")
  # "this one lets you use external frame start triggers"
  # "C:\\Users\\Public\\Documents\\National Instruments\\NI-IMAQdx\\Data\\XML\nalso programming manual"
  n1 = local read "Exposure time (us)"() -> (w11:dbl)
  n2 = call <vilib>:"IMAQdx Open Camera.vi"("Session In"="Session In") -> ("error out"=w6:errorcluster, "Session Out"=w7:T3)  [unwired: 9 in]
  n3 = property on="Exposure time (us)" class="DigNum (strict)"("Val(Sgnl)"=w11) -> (error out=w5:errorcluster)  [unwired: 2 in, 1 out]
  n4 = call <vilib>:"IMAQdx Configure Grab.vi"("error in"=w6, "Session In"=w7) -> ("error out"=w12:errorcluster, "Session Out"=w13:T3)  [unwired: 8 in]
  n5 = call "IMAQ Create"("Image Name"="untitled", "Image Type"=w9) -> ("New Image"=w8:T5)  [unwired: 3 in, 1 out]
  n6 = while {
    tunnel: w13 -> [w33]
    tunnel: [w32] -> w3
    tunnel: w12 -> [w24]
    tunnel: w8 -> [w23]
    tunnel: w5 -> [_]
    tunnel: ["save?"] -> w4
    tunnel: [w17] -> w2
    tunnel: [w16] -> w1
    stop <- "stop" stop-if-true
    n7 = event shown="[0] \"external frame start triggers?\", \"Height\", \"Width\", \"Offset X\", \"Offset Y\", \"Exposure time (us)\": Value Change" {
      selector: _ -> [_ _]
      dyn-events: _ -> [_ _]
      timeout: 10 -> [_ _]
      tunnel: w33 -> [w37 w103]
      tunnel: w24 -> [w36 w104]
      tunnel: [w39 w103] -> w27
      tunnel: [w38 w104] -> w26
      event "external frame start triggers?", "Height", "Width", "Offset X", "Offset Y", "Exposure time (us)": Value Change {
        n8 = event-data() -> ()  [unwired: 1 in, 6 out]
        n9 = flat-sequence {
          tunnel: w36 -> [w50]
          tunnel: w37 -> [w51]
          tunnel: [w51] -> w35
          tunnel: [w50] -> w34
          tunnel: [w101] -> w39
          tunnel: [w100] -> w38
          tunnel: w35 -> [w98]
          tunnel: w34 -> [w97]
          frame #0 {
            n10 = local read "Offset X"() -> (w48:i64)
            n11 = local read "Offset Y"() -> (w47:i64)
            n12 = local read "Height"() -> (w46:i64)
            n13 = call "coerce width height.vi"("Offset Y"=w47, "Offset X"=w48) -> ("max height"=w49:i64, "max width"=w40:i64)  [unwired: 8 in]
            n14 = local read "Width"() -> (w45:i64)
            n15 = property on="Width" class="Slide (strict)"("Maximum"=w40) -> ()  [unwired: 2 in, 2 out]
            n16 = In Range and Coerce(upper limit=w49, x=w46, lower limit=i64 4) -> (coerced(x)=w41:i64)  [unwired: 1 out]
            n17 = property on="Height" class="Slide (strict)"("Maximum"=w49) -> ()  [unwired: 2 in, 2 out]
            n18 = local write "Height"(w41) -> ()
            n19 = In Range and Coerce(upper limit=w40, x=w45, lower limit=i64 4) -> (coerced(x)=w42:i64)  [unwired: 1 out]
            n20 = property on="Intensity Graph" class="IntGraph (strict)"("YScale.Maximum"=w41) -> ()  [unwired: 2 in, 2 out]
            n21 = local write "Width"(w42) -> ()
            n22 = property on="Intensity Graph" class="IntGraph (strict)"("XScale.Maximum"=w42) -> ()  [unwired: 2 in, 2 out]
          }
          frame #1 {
            # "ReverseY true\nmake origin in lower left"
            # "turn off frame burst trigger"
            # "trigger line debounce time\nin us"
            # "4 frames"
            # "pick source\nline3 = 3, line4 = 4"
            # "triggers off = 0, on = 1"
            # "FrameBurstStart = 0\nFrameStart = 1"
            n23 = call <vilib>:"IMAQdx Unconfigure Acquisition.vi"("error in"=w97, "Session In"=w98) -> ("error out"=w94:errorcluster, "Session Out"=w95:T3)  [unwired: 8 in]
            n24 = call <vilib>:"IMAQdx Enumerate Attributes.vi"("error in"=w94, "Session In"=w95) -> ("error out"=w92:errorcluster, "Attribute Information Array"=→"Attribute Information Array":T2, "Session Out"=w93:T3)  [unwired: 7 in]
            n25 = local read "Exposure time (us)"() -> (w90:dbl)
            n26 = local read "Height"() -> (w91:i64)
            n27 = local read "Offset X"() -> (w86:i64)
            n28 = local read "Width"() -> (w89:i64)
            n29 = local read "Offset Y"() -> (w84:i64)
            n30 = property class="IMAQdx"(reference=w93, error in=w92, "ActiveAttribute"="CameraAttributes::AcquisitionControl::ExposureTime", "ValueDBL"=w90, "ActiveAttribute"="CameraAttributes::ImageFormatControl::Height", "ValueI64"=w91, "ActiveAttribute"="CameraAttributes::ImageFormatControl::Width", "ValueI64"=w89, "ActiveAttribute"="CameraAttributes::ImageFormatControl::OffsetX", "ValueI64"=w86, "ActiveAttribute"="CameraAttributes::ImageFormatControl::OffsetY", "ValueI64"=w84, "ActiveAttribute"="CameraAttributes::ImageFormatControl::ReverseY", "ValueBool"=TRUE) -> (reference out=w76:T3)  [unwired: 1 out]
            n31 = Select(t=i64 1 ("ValueI64"), s="external frame start triggers?", f=i64 0 ("ValueI64")) -> (s? t:f=w73:i64)
            n32 = property class="IMAQdx"(reference=w76, "ActiveAttribute"="CameraAttributes::AcquisitionControl::TriggerSelector", "ValueU32"=i64 1 ("ValueI64"), "ActiveAttribute"="CameraAttributes::AcquisitionControl::TriggerMode", "ValueU32"=w73, "ActiveAttribute"="CameraAttributes::AcquisitionControl::TriggerSource", "ValueU32"=i64 4 ("ValueI64"), "ActiveAttribute"="CameraAttributes::AcquisitionControl::AcquisitionBurstFrameCount", "ValueU32"=i64 3 ("ValueI64"), "ActiveAttribute"="CameraAttributes::DigitalIOControl::LineDebouncerTime", "ValueU32"=u32 0, "ActiveAttribute"="CameraAttributes::AcquisitionControl::TriggerSelector", "ValueU32"=i64 0 ("ValueI64"), "ActiveAttribute"="CameraAttributes::AcquisitionControl::TriggerMode", "ValueU32"=i64 0 ("ValueI64"), "ActiveAttribute"="CameraAttributes::AcquisitionControl::ResultingFrameRate") -> (reference out=w60:T3, "ValueDBL"=w62:dbl)  [unwired: 1 in, 1 out]
            "frame rate (Hz)" <- w62
            n33 = Reciprocal(x=w62) -> (1/x=→"frame time (s)":dbl)
            n34 = property class="IMAQdx"(reference=w60, "ActiveAttribute"="CameraAttributes::RemoveParameterLimitControl::RemoveParameterLimitSelector", "ValueU32"=u32 0, "ActiveAttribute"="CameraAttributes::RemoveParameterLimitControl::RemoveParameterLimit", "ValueBool"=TRUE) -> (reference out=w57:T3)  [unwired: 1 in, 1 out]
            n35 = property class="IMAQdx"(reference=w57, "ActiveAttribute"="CameraAttributes::AnalogControl::Gain", "ValueDBL"=0.0) -> (reference out=w56:T3)  [unwired: 1 in, 1 out]
            n36 = call <vilib>:"IMAQdx Configure Grab.vi"("Session In"=w56) -> ("error out"=w100:errorcluster, "Session Out"=w101:T3)  [unwired: 9 in]
          }
        }
      }
      event Timeout {
        n37 = event-data() -> ()  [unwired: 1 in, 2 out]
      }
    }
    n38 = call <vilib>:"IMAQdx Grab2.vi"("error in"=w26, "Image In"=w23, "Session In"=w27) -> ("error out"=w29:errorcluster, "Buffer Number Out"=w31:u32, "Image Out"=w17:T5, "Session Out"=w25:T3)  [unwired: 5 in]
    n39 = call <vilib>:"IMAQdx Get Image Data.vi"("Buffer Number Mode (Next)"=IMAQdx_Buffer_Number_Mode."Last", "error in"=w29, "Buffer Number In"=w31, "Session In"=w25) -> ("Image Data Array"=w20:u8[], "Session Out"=w32:T3)  [unwired: 4 in, 2 out]
    n40 = Array Max & Min(array=w20) -> (max value=→"max value":u8)  [unwired: 3 out]
    n41 = local read "Height"() -> (w21:i64)
    n42 = local read "Width"() -> (w22:i64)
    n43 = call-poly "convert 1D image array to 2D image - polymorphic.vi"("Height"=w21, "Width"=w22, "Image Data Array"=w20) -> ("Intensity Graph"=w16:u8[][])  [unwired: 8 in]
    "Intensity Graph" <- w16
  }
  n44 = call <vilib>:"IMAQdx Close Camera.vi"("Session In"=w3) -> ()  [unwired: 10 in, 1 out]
  n45 = case shown="True" w4 {
    tunnel: w2 -> [_ w115]
    tunnel: w1 -> [_ w108]
    frame False {
    }
    frame True {
      w114 = u32 0 items=["Horizontal", "Vertical", "Central", "1st Diagonal", "2nd Diagonal"] ("Type of Symmetry")
      # "convention of origin always in bottom left corner"
      n46 = local write "save?"(FALSE ("save?")) -> ()
      n47 = Concatenate Strings("filename", ".jpg" ("string")) -> (w118:string)
      n48 = Concatenate Strings("filename", ".csv" ("string")) -> (w110:string)
      n49 = call "IMAQ Symmetry"("Type of Symmetry"=w114, "Image Src"=w115) -> ("Image Dst Out"=w116:T5)  [unwired: 3 in, 1 out]
      n50 = Build Path(base path="path", name or relative path=w118) -> (appended path=w117:path)
      n51 = Build Path(base path="path", name or relative path=w110) -> (appended path=w109:path)
      n52 = call-poly "IMAQ Write File 2"("File Path"=w117, "Image"=w116) -> ()  [unwired: 8 in, 2 out]
      n53 = call-poly <vilib>:"Write Delimited Spreadsheet.vi"("file path (dialog if empty)"=w109, "2D data"=w108, "append to file? (new file:F)"=FALSE, "transpose? (no:F)"=TRUE) -> ()  [unwired: 10 in, 2 out]
    }
  }
